vi "OPEN_ALL_RELAYS.vi"   [LabVIEW 2019]
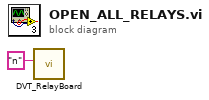
[diagram p0: block diagram]
diagram:
  n1 = call "DVT_RelayBoard.vi"("write buffer"="n") -> ()  [unwired: 3 in, 3 out]
